vi "function1 new.vi"   [LabVIEW 2016, in "Test2.lvrbt"]
uses:
  Test2.lvrbt
  <vilib>/NXT/Block Support/NXT_InputPort.ctl
  <vilib>/NXT/Hardware/Plugins/Tetrix DC Motor/TetrixDCMotorAddress.ctl
  <vilib>/NXT/NXTIO Xnodes/NXTIONodeSubVIs/TETRIX IO Move DC Motors.vi
  <vilib>/NXT/Dual Mode Library/Waits/Wait_EV3_Ultrasonic_Centimeter_Closer.vi
  <vilib>/NXT/NXTIO Xnodes/NXTIONodeSubVIs/TETRIX IO Stop DC Motors.vi
  <vilib>/NXT/Dual Mode Library/Waits/Wait_Num.vi
  <vilib>/NXT/Dual Mode Library/Waits/Wait_EV3_Ultrasonic_Centimeters_Further.vi
  <vilib>/NXT/Subs/LVHSConnector.ctl
  <vilib>/NXT/NXTIO Xnodes/AddressXNode/NXTIOAddress.xnode
  <vilib>/NXT/NXTIO Xnodes/NXTIOXNode/NXTIO.xnode
  <vilib>/NXT/LegoClasses/BrickReference/BrickReference.lvclass
types:
  T1 = typedef "NXT_InputPort.ctl" = u32
  T2 = typedef "TetrixDCMotorAddress.ctl" = i32
  T3 = typedef "LVHSConnector.ctl" = refnum<class "BrickReference.lvclass">
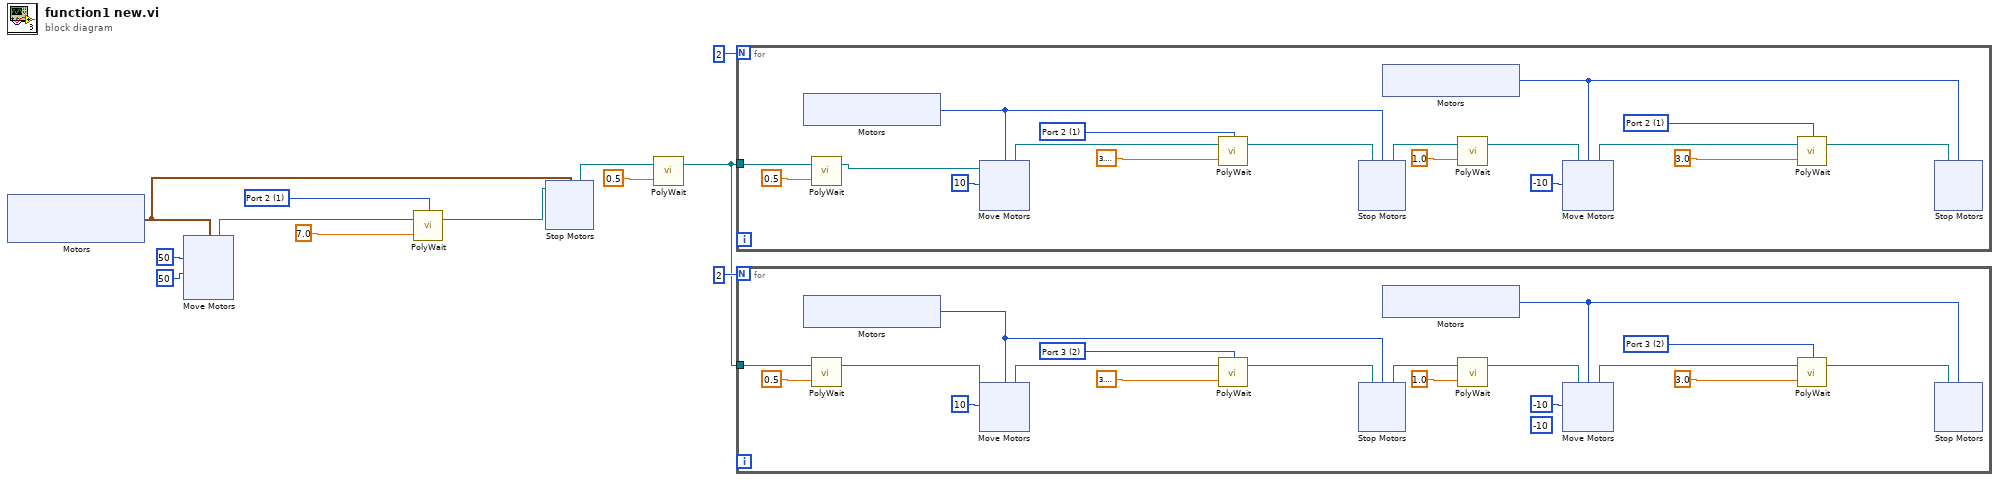
[diagram p0: block diagram]
diagram:
  w6 = T1 1 items=["Port 1", "Port 2", "Port 3", "Port 4"] ("Port (Port 1)")
  n1 = xnode "Motors"() -> ("Motor"=w7:cluster{"TetrixDCMotor":T2, "TetrixDCMotor":T2})
  n2 = xnode "Move Motors"("Power/Speed 2"=i8 50, "Power/Speed 1"=i8 50, "Motors"=w7) -> ("NXT/EV3"=w10:T3)  [unwired: 1 in]
  n3 = call-poly <vilib>:"PolyWait.vi"("Centimeters (40)"=sgl 7.0, "NXT/EV3"=w10, "Port (Port 1)"=w6) -> ("NXT/EV3"=w8:T3)  [unwired: 1 in]
  n4 = xnode "Stop Motors"("Motors"=w7, "NXT/EV3"=w8) -> ("NXT/EV3"=w3:T3)
  n5 = call-poly <vilib>:"PolyWait.vi"("Time (1 sec)"=sgl 0.5, "NXT/EV3"=w3) -> ("NXT/EV3"=w1:T3)  [unwired: 2 in]
  n6 = for {
    N: 2 -> [_]
    tunnel: w1 -> [w13]
    w18 = T1 1 items=["Port 1", "Port 2", "Port 3", "Port 4"] ("Port (Port 1)")
    w25 = T1 1 items=["Port 1", "Port 2", "Port 3", "Port 4"] ("Port (Port 1)")
    n7 = xnode "Motors"() -> ("Motor"=w26:T2)
    n8 = call-poly <vilib>:"PolyWait.vi"("Time (1 sec)"=sgl 0.5, "NXT/EV3"=w13) -> ("NXT/EV3"=w14:T3)  [unwired: 2 in]
    n9 = xnode "Move Motors"("Power/Speed 1"=i8 10, "Motors"=w26, "NXT/EV3"=w14) -> ("NXT/EV3"=w29:T3)
    n10 = call-poly <vilib>:"PolyWait.vi"("Centimeters (40)"=sgl 3.2, "NXT/EV3"=w29, "Port (Port 1)"=w25) -> ("NXT/EV3"=w27:T3)  [unwired: 1 in]
    n11 = xnode "Stop Motors"("Motors"=w26, "NXT/EV3"=w27) -> ("NXT/EV3"=w23:T3)
    n12 = xnode "Motors"() -> ("Motor"=w16:T2)
    n13 = call-poly <vilib>:"PolyWait.vi"("Time (1 sec)"=sgl 1.0, "NXT/EV3"=w23) -> ("NXT/EV3"=w22:T3)  [unwired: 2 in]
    n14 = xnode "Move Motors"("Power/Speed 1"=i8 -10, "Motors"=w16, "NXT/EV3"=w22) -> ("NXT/EV3"=w20:T3)
    n15 = call-poly <vilib>:"PolyWait.vi"("Centimeters (50)"=sgl 3.0, "NXT/EV3"=w20, "Port (Port 1)"=w18) -> ("NXT/EV3"=w17:T3)  [unwired: 1 in]
    n16 = xnode "Stop Motors"("Motors"=w16, "NXT/EV3"=w17) -> ()  [unwired: 1 out]
  }
  n17 = for {
    N: 2 -> [_]
    tunnel: w1 -> [w57]
    w62 = T1 2 items=["Port 1", "Port 2", "Port 3", "Port 4"] ("Port (Port 1)")
    (unwired) i8 -10 ("Power/Speed 2")
    w69 = T1 2 items=["Port 1", "Port 2", "Port 3", "Port 4"] ("Port (Port 1)")
    n18 = xnode "Motors"() -> ("Motor"=w70:T2)
    n19 = call-poly <vilib>:"PolyWait.vi"("Time (1 sec)"=sgl 0.5, "NXT/EV3"=w57) -> ("NXT/EV3"=w58:T3)  [unwired: 2 in]
    n20 = xnode "Move Motors"("Power/Speed 1"=i8 10, "Motors"=w70, "NXT/EV3"=w58) -> ("NXT/EV3"=w73:T3)
    n21 = call-poly <vilib>:"PolyWait.vi"("Centimeters (40)"=sgl 3.2, "NXT/EV3"=w73, "Port (Port 1)"=w69) -> ("NXT/EV3"=w71:T3)  [unwired: 1 in]
    n22 = xnode "Stop Motors"("Motors"=w70, "NXT/EV3"=w71) -> ("NXT/EV3"=w67:T3)
    n23 = xnode "Motors"() -> ("Motor"=w60:T2)
    n24 = call-poly <vilib>:"PolyWait.vi"("Time (1 sec)"=sgl 1.0, "NXT/EV3"=w67) -> ("NXT/EV3"=w66:T3)  [unwired: 2 in]
    n25 = xnode "Move Motors"("Power/Speed 1"=i8 -10, "Motors"=w60, "NXT/EV3"=w66) -> ("NXT/EV3"=w64:T3)
    n26 = call-poly <vilib>:"PolyWait.vi"("Centimeters (50)"=sgl 3.0, "NXT/EV3"=w64, "Port (Port 1)"=w62) -> ("NXT/EV3"=w61:T3)  [unwired: 1 in]
    n27 = xnode "Stop Motors"("Motors"=w60, "NXT/EV3"=w61) -> ()  [unwired: 1 out]
  }
